vi "Read bombed.vi"(8 "error in (no error)":errorcluster, 11 "BombedWall in":refnum<class "BombedWall.lvclass">) -> (0 "error out":errorcluster, 2 "bombed":bool, 3 "BombedWall out":refnum<class "BombedWall.lvclass">)   [LabVIEW 2016, in "BombedWall.lvclass"]
uses:
  BombedWall.lvclass
  BombedWall.lvclass/BombedWall.ctl
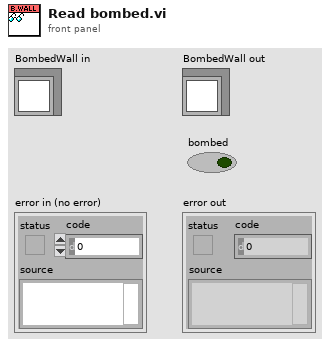
[diagram p1: front panel]
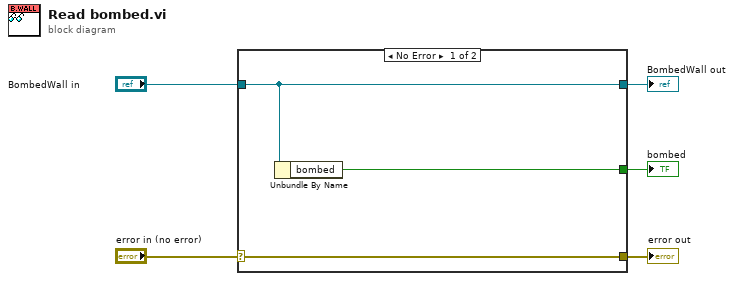
[diagram p0: block diagram]
diagram:
  n1 = case shown="No Error" "error in (no error)" {
    selector: "error in (no error)" -> [w8 w9]
    tunnel: [w8 w9] -> w4
    tunnel: [w7 w10] -> w2
    tunnel: "BombedWall in" -> [w7 w10]
    tunnel: [w6 _] -> w1
    frame No Error {
      n2 = Unbundle By Name(w7) -> ("bombed"=w6:bool)
    }
    frame Error {
    }
  }
  "error out" <- w4
  "BombedWall out" <- w2
  "bombed" <- w1
